vi "Reset.vi"(8 "error in (no error)":errorcluster, 11 "SR3XXX in":refnum<class "SR3XXX HVPS.lvclass">) -> (0 "error out":errorcluster, 3 "SR3XXX out":refnum<class "SR3XXX HVPS.lvclass">)   [LabVIEW 2014, in "SR3XXX HVPS.lvclass"]
doc: "The *RST common command resets the power supply to its default configuration. It is the same as holding the [CLR] button depressed at power on."
uses:
  SR3XXX HVPS.lvclass
  reusable/Session APIs/Serial/Typedefs/Session Handle.ctl
  reusable/Session APIs/Serial/Serial Session.lvclass
  Base/Session HVPS.lvclass/Session HVPS.ctl
  Base/Read hSession.vi
  reusable/Session APIs/Serial/Public/Asynchronous Write.vi
  <userlib>/_Session Fwk/Session - Root.lvclass
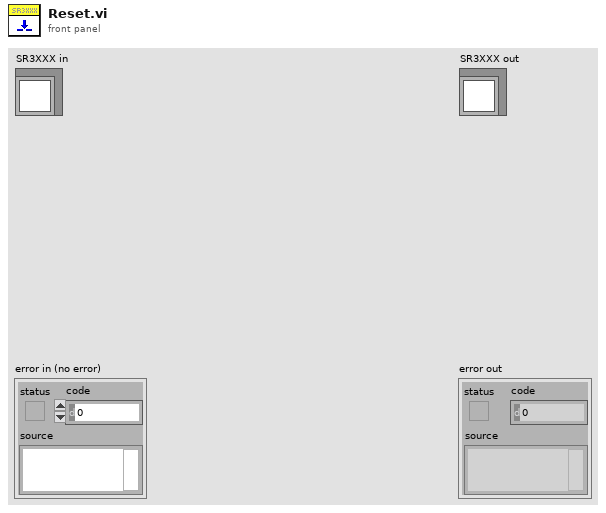
[diagram p1: front panel]
types:
  T1 = typedef "Serial Session.lvclass/Session Handle.ctl" = refnum<data-value>
  T2 = typedef "Session - Root.lvclass/Session Handle.ctl" = refnum<data-value>
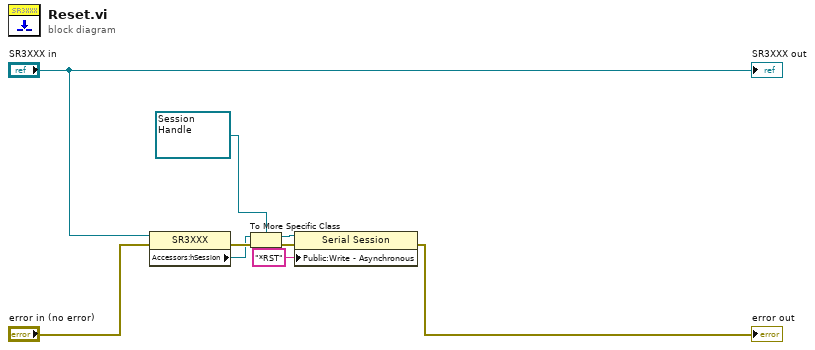
[diagram p0: block diagram]
diagram:
  n1 = property class="SR3XXX"(reference="SR3XXX in", error in="error in (no error)") -> (error out=w8:errorcluster, "Accessors:hSession"=w7:T2)  [unwired: 1 out]
  n2 = To More Specific Class(target class=T1 refnum ("Session Handle"), reference=w7, error in=w8) -> (specific class reference=w5:T1, error out=w9:errorcluster)
  n3 = property class="Serial Session"(reference=w5, error in=w9, "Public:Write - Asynchronous"="*RST" ("Write - Asynchronous")) -> (error out=→"error out":errorcluster)  [unwired: 1 out]
  "SR3XXX out" <- "SR3XXX in"
